vi "Radau5_E Norm.vi"(11 "Vector in":dbl[](array[numeric])) -> (3 "Norm output":dbl)   [LabVIEW 2020, in "NI_DAE.lvlib"]
uses:
  <vilib>/gmath/NI_DAE.lvlib
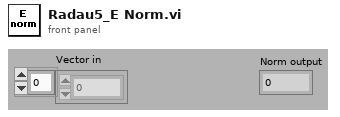
[diagram p1: front panel]
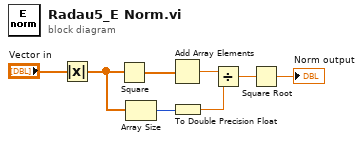
[diagram p0: block diagram]
diagram:
  n1 = Absolute Value(x="Vector in") -> (abs(x)=w1:dbl[])
  n2 = Square(x=w1) -> (x^2=w8:dbl[])
  n3 = Array Size(array=w1) -> (size(s)=w5:i32)
  n4 = Add Array Elements(numeric array=w8) -> (sum=w7:dbl)
  n5 = To Double Precision Float(number=w5) -> (double precision float=w6:dbl)
  n6 = Divide(x=w7, y=w6) -> (x/y=w4:dbl)
  n7 = Square Root(x=w4) -> (sqrt(x)=→"Norm output":dbl)
